vi "SVT Peak Level.vi"   [LabVIEW 2017]
doc: "Computes the peak level of <B>scaled signal [EU]</B>. You can use this polymorphic VI to compute the peak level for a single channel or for N channels. The data type you wire to the <B>scaled signal [EU]</B> input determines the polymorphic instance to use."
uses:
  <vilib>/addons/Sound and Vibration/svt_Level/SoundVib_VibrationLevel.lvlib
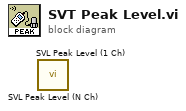
[diagram p0: block diagram]
diagram:
  n1 = call <vilib>:"SVL Peak Level (N Ch).vi"() -> ()  [unwired: 9 in, 3 out]
  n2 = call <vilib>:"SVL Peak Level (1 Ch).vi"() -> ()  [unwired: 9 in, 3 out]
